vi "PCP com S&E serialized.vi"(0 "Loop ID in":u16, 2 "Periodic(F)":bool, 7 "Serialized Receive":string, 9 "Serialized send":string, 11 "error in (no error)":errorcluster, 13 "Reply":bool) -> (4 "Loop ID out":u16, 15 "error out":errorcluster)   [LabVIEW 2011]
uses:
  Application Structure/E&S Note ID.ctl
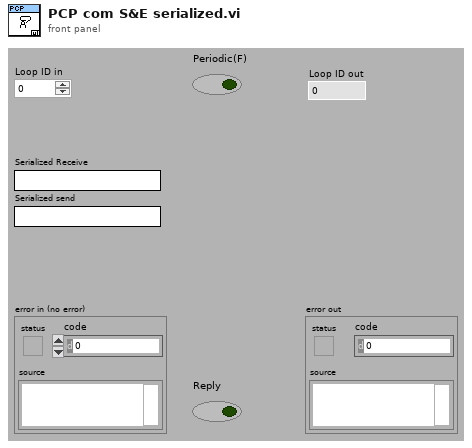
[diagram p1: front panel]
types:
  T1 = typedef "E&S Note ID.ctl" = enum16{"Program Started", "Program terminated", "User Changed", "General information"}
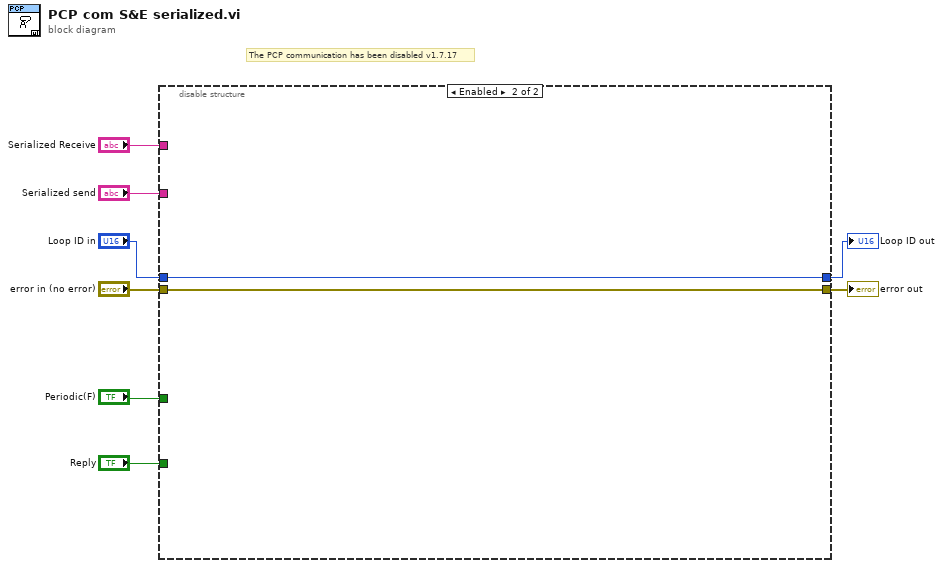
[diagram p0: block diagram]
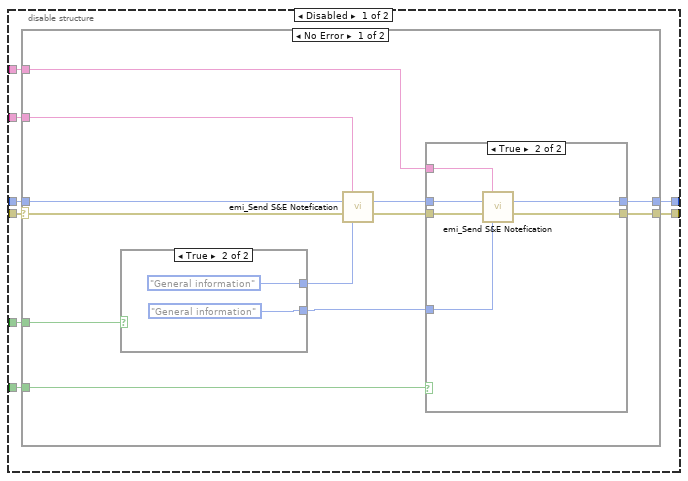
[diagram p2: hidden frame]
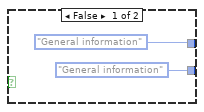
[diagram p4: hidden frame]
diagram:
  # "The PCP communication has been disabled v1.7.17"
  n1 = disable-structure shown="Enabled" {
    disable-tunnel: "Serialized send" -> [w16 _]
    disable-tunnel: "Loop ID in" -> [w15 w44]
    disable-tunnel: "Periodic(F)" -> [w14 _]
    disable-tunnel: [w13 w44] -> w5
    disable-tunnel: [w12 w43] -> w4
    disable-tunnel: "Reply" -> [w11 _]
    disable-tunnel: "Serialized Receive" -> [w10 _]
    disable-tunnel: "error in (no error)" -> [w9 w43]
    frame Disabled {
      n2 = case shown="No Error" w9 {
        selector: w9 -> [w18 w42]
        tunnel: w16 -> [w28 _]
        tunnel: w15 -> [w27 w41]
        tunnel: w14 -> [w26 _]
        tunnel: [w23 w41] -> w13
        tunnel: [w22 w42] -> w12
        tunnel: w11 -> [w21 _]
        tunnel: w10 -> [w20 _]
        frame No Error {
          n3 = case shown="True" w26 {
            tunnel: [E&S_Note_ID."General information" ("E&S note ID") E&S_Note_ID."General information" ("E&S note ID")] -> w17
            tunnel: [E&S_Note_ID."General information" ("E&S note ID") E&S_Note_ID."General information" ("E&S note ID")] -> w19
            frame False {
            }
            frame True {
            }
          }
          n4 = call "emi_Send S&E Notefication.vi"("Note(\"\")"=w28, "Loop ID in(No ID)"=w27, "error in (no error)"=w18, "Loc Sub ID/Note ID"=w17) -> ("Loop ID out"=w24:u16, "error out"=w25:errorcluster)  [unwired: 10 in]
          n5 = case shown="True" w21 {
            tunnel: w25 -> [w29 w36]
            tunnel: w24 -> [w30 w35]
            tunnel: [w30 w34] -> w23
            tunnel: [w29 w33] -> w22
            tunnel: w20 -> [_ w32]
            tunnel: w19 -> [_ w31]
            frame False {
            }
            frame True {
              n6 = call "emi_Send S&E Notefication.vi"("Note(\"\")"=w32, "Loop ID in(No ID)"=w35, "error in (no error)"=w36, "Loc Sub ID/Note ID"=w31) -> ("Loop ID out"=w34:u16, "error out"=w33:errorcluster)  [unwired: 10 in]
            }
          }
        }
        frame Error {
        }
      }
    }
    frame Enabled {
    }
  }
  "error out" <- w4
  "Loop ID out" <- w5
